vi "mobility_subvi.vi"(0 "Path":path, 9 "NumPts":dbl=5.0, 11 "Row Start":dbl=20.0) -> (1 "Dielectric (d)":dbl, 2 "Capacitance (C)":dbl, 3 "Index":dbl, 4 "XY Graph":cluster{dbl[], dbl[]}[](graph), 6 "Length":dbl, 8 "Vt":dbl, 10 "Width":dbl, 12 "Table Control":string[][](table), 13 "Table Control 2":string[][](table), 14 "Recorded":cluster{"Vt":dbl, "STS":dbl, "On/Off":dbl}, 15 "Mobility":dbl)   [LabVIEW 2011]
uses:
  <vilib>/Utility/file.llb/Read From Spreadsheet File (string).vi
  <vilib>/Analysis/NI_AALPro.lvlib
panel:
  out "Numeric":dbl
  out "String":string
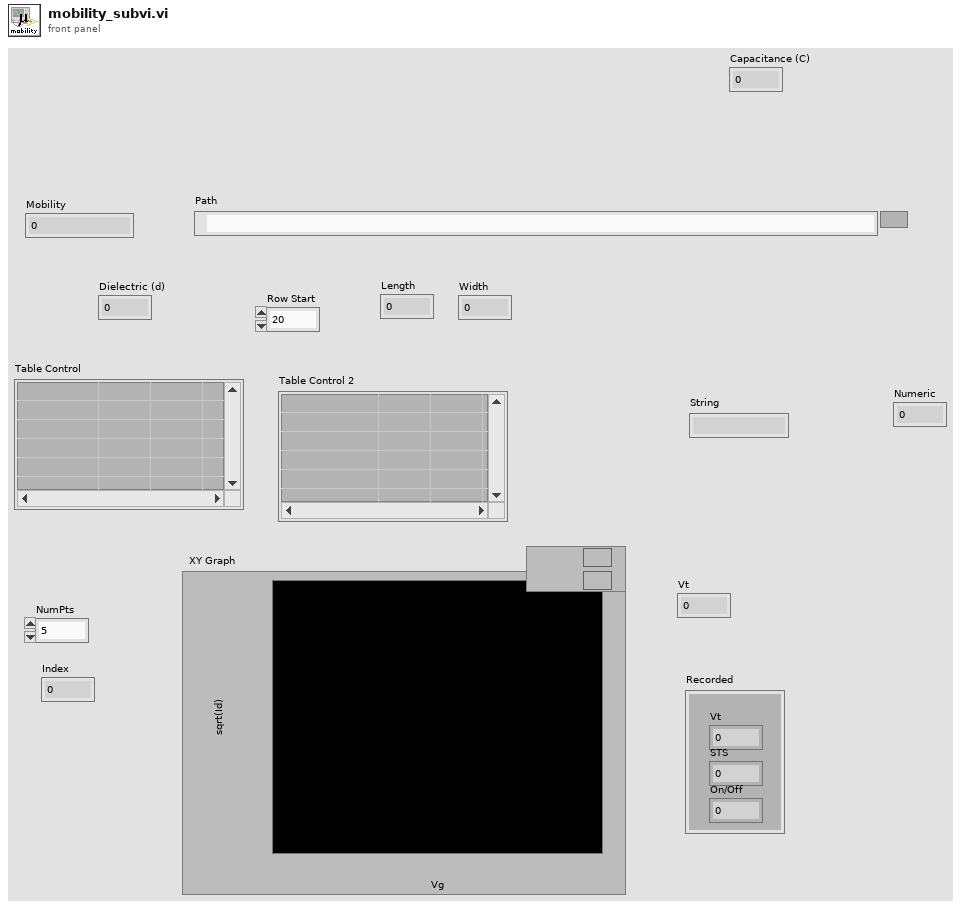
[diagram p1: front panel]
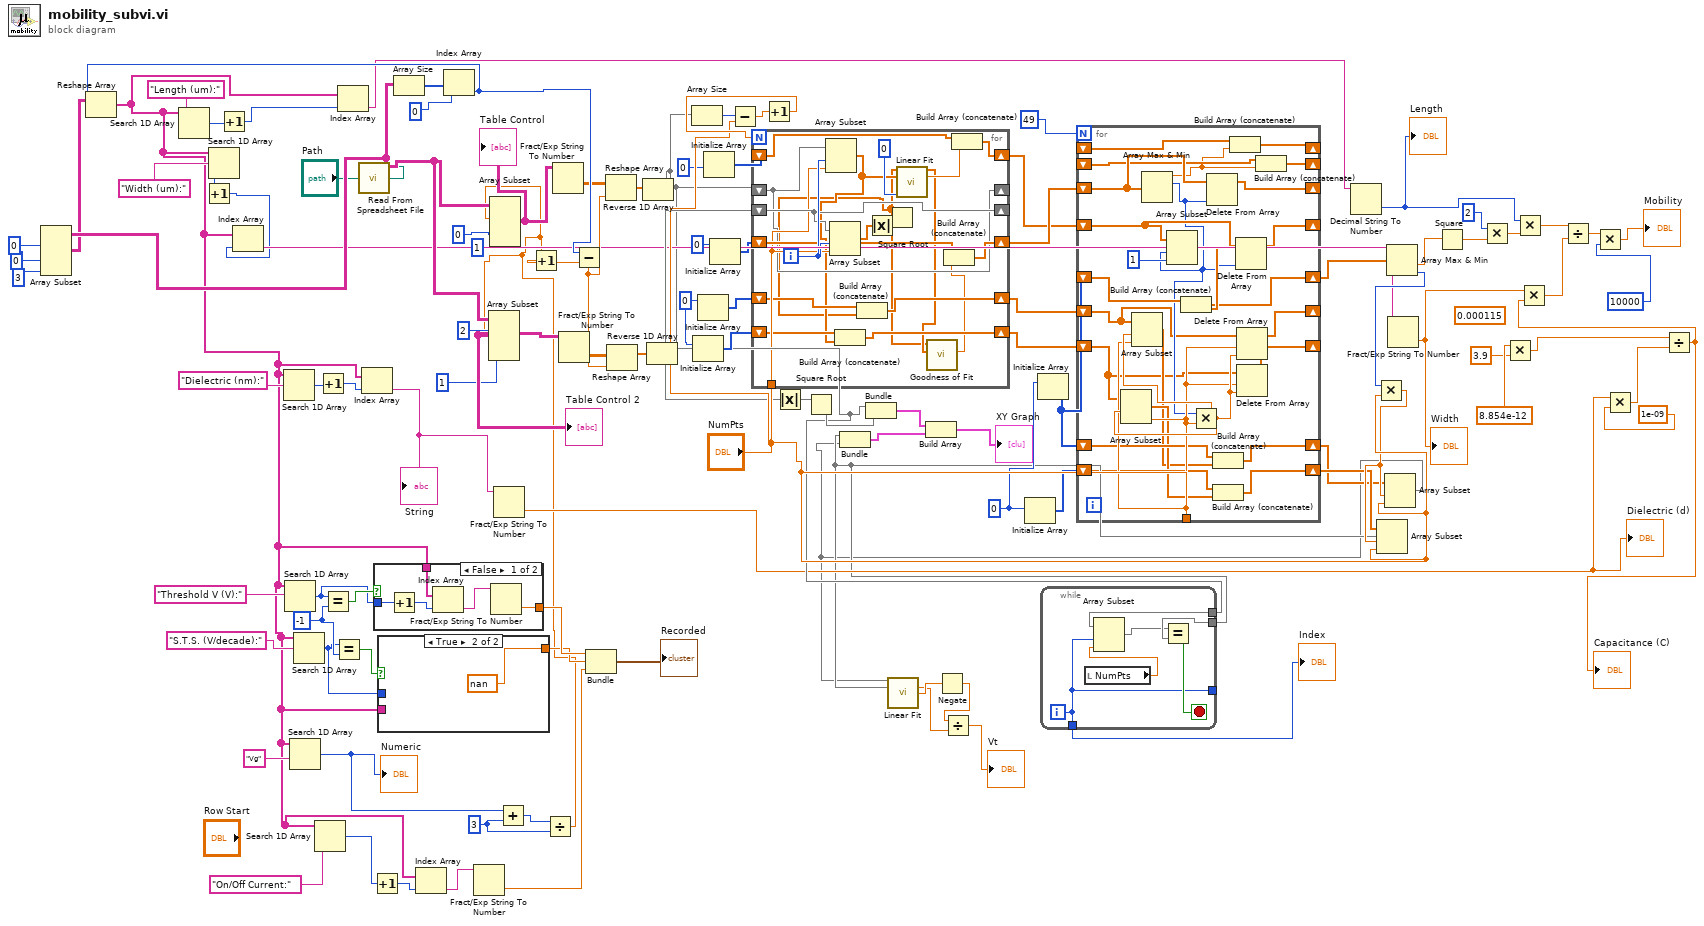
[diagram p0: block diagram]
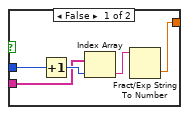
[diagram p2: hidden frame]
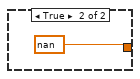
[diagram p3: hidden frame]
diagram:
  w9 = 3
  w20 = -1
  w97 = 0
  w88 = 0
  (unwired) 0.000115
  n1 = call-poly <vilib>:"Read From Spreadsheet File.vi"("file path (dialog if empty)"="Path") -> ("all rows"=w76:string[][])  [unwired: 6 in, 4 out]
  n2 = Array Subset(array=w76, index (row)=0, index (col)=0, length (col)=3) -> (w72:string[][])  [unwired: 1 in]
  n3 = Array Size(array=w76) -> (size(s)=w78:i32[])
  n4 = Index Array(array=w78, index=0) -> (element=w105:i32)
  n5 = Reshape Array(w72, w105) -> (w3:string[])
  n6 = Search 1D Array(1D array=w3, element="Length (um):") -> (index of element=w62:i32)  [unwired: 1 in]
  n7 = Search 1D Array(1D array=w3, element="Width (um):") -> (index of element=w63:i32)  [unwired: 1 in]
  n8 = Increment(x=w63) -> (x+1=w69:i32)
  n9 = Increment(x=w62) -> (x+1=w66:i32)
  n10 = Index Array(array=w3, index=w69) -> (element=w70:string)
  n11 = Search 1D Array(1D array=w3, element="Dielectric (nm):") -> (index of element=w32:i32)  [unwired: 1 in]
  n12 = Search 1D Array(1D array=w3, element="Threshold V (V):") -> (index of element=w17:i32)  [unwired: 1 in]
  n13 = Search 1D Array(1D array=w3, element="Vg") -> (index of element=w11:i32)  [unwired: 1 in]
  "Numeric" <- w11
  n14 = Search 1D Array(1D array=w3, element="S.T.S. (V/decade):") -> (index of element=w16:i32)  [unwired: 1 in]
  n15 = Search 1D Array(1D array=w3, element="On/Off Current:") -> (index of element=w4:i32)  [unwired: 1 in]
  n16 = Increment(x=w32) -> (x+1=w31:i32)
  n17 = Equal?(x=w17, y=w20) -> (x = y?=w19:bool)
  n18 = Equal?(x=w16, y=w20) -> (x = y?=w18:bool)
  n19 = Index Array(array=w3, index=w66) -> (element=w67:string)
  n20 = Index Array(array=w3, index=w31) -> (element=w30:string)
  "String" <- w30
  n21 = Increment(x=w4) -> (x+1=w5:i32)
  n22 = case shown="False" w19 {
    tunnel: w17 -> [w114 _]
    tunnel: w3 -> [w113 _]
    tunnel: [w111 nan] -> w15
    frame False {
      n23 = Increment(x=w114) -> (x+1=w115:i32)
      n24 = Index Array(array=w113, index=w115) -> (element=w112:string)
      n25 = Fract/Exp String To Number(string=w112) -> (number=w111:dbl)  [unwired: 3 in, 1 out]
    }
    frame True {
    }
  }
  n26 = case shown="True" w18 {
    tunnel: w16 -> [w120 _]
    tunnel: w3 -> [w119 _]
    tunnel: [w117 nan] -> w14
    frame False {
      n27 = Increment(x=w120) -> (x+1=w121:i32)
      n28 = Index Array(array=w119, index=w121) -> (element=w118:string)
      n29 = Fract/Exp String To Number(string=w118) -> (number=w117:dbl)  [unwired: 3 in, 1 out]
    }
    frame True {
    }
  }
  n30 = Index Array(array=w3, index=w5) -> (element=w6:string)
  n31 = Fract/Exp String To Number(string=w6) -> (number=w2:dbl)  [unwired: 3 in, 1 out]
  n32 = Fract/Exp String To Number(string=w30) -> (number=w29:dbl)  [unwired: 3 in, 1 out]
  "Dielectric (d)" <- w29
  n33 = Add(x=w11, y=w9) -> (x+y=w10:i32)
  n34 = Divide(x=w10, y=w9) -> (x/y=w8:dbl)
  n35 = Array Subset(array=w76, index (row)=w8, index (col)=2, length (col)=1) -> (w55:string[][])  [unwired: 1 in]
  "Table Control 2" <- w55
  n36 = Array Subset(array=w76, index (row)=w8, index (col)=0, length (col)=1) -> (w54:string[][])  [unwired: 1 in]
  "Table Control" <- w54
  n37 = Increment(x=w8) -> (x+1=w106:dbl)
  n38 = Fract/Exp String To Number(string=w54) -> (number=w56:dbl[][])  [unwired: 3 in, 1 out]
  n39 = Fract/Exp String To Number(string=w55) -> (number=w57:dbl[][])  [unwired: 3 in, 1 out]
  n40 = Subtract(x=w105, y=w106) -> (x-y=w107:dbl)
  n41 = Bundle(w15, w14, w2) -> (→"Recorded":cluster{dbl, dbl, dbl})  [unwired: 1 in]
  n42 = Reshape Array(w56, w107) -> (w93:dbl[])
  n43 = Reshape Array(w57, w107) -> (w94:dbl[])
  n44 = Reverse 1D Array(array=w93) -> (reversed array=w35:dbl[])
  n45 = Reverse 1D Array(array=w94) -> (reversed array=w95:dbl[])
  n46 = Array Size(array=w35) -> (size(s)=w48:i32)
  n47 = Initialize Array(w88) -> (w90:i32[])  [unwired: 1 in]
  n48 = Initialize Array(w88) -> (w89:i32[])  [unwired: 1 in]
  n49 = Initialize Array(0) -> (w49:i32[])  [unwired: 1 in]
  n50 = Initialize Array(0) -> (w50:i32[])  [unwired: 1 in]
  n51 = Subtract(x=w48, y="NumPts") -> (x-y=w109:dbl)
  n52 = Increment(x=w109) -> (x+1=w110:dbl)
  n53 = for {
    N: w110 -> [_]
    shift-right: [w127] -> _
    shift-left: w35 -> [w127]
    shift-right: [w136] -> _
    shift-left: w95 -> [w136]
    shift-right: [w140] -> w59
    shift-left: w49 -> [w139]
    shift-right: [w138] -> w79
    shift-left: w50 -> [w137]
    tunnel: "NumPts" -> [w132]
    shift-right: [w130] -> w91
    shift-left: w89 -> [w131]
    shift-right: [w128] -> w92
    shift-left: w90 -> [w129]
    i -> [w142]
    n54 = Array Subset(array=w127, index=w142, length=w132) -> (w126:dbl[])
    n55 = Array Subset(array=w136, index=w142, length=w132) -> (w135:dbl[])
    n56 = Build Array (concatenate)(w129, w126) -> (w128:dbl[])
    n57 = Absolute Value(x=w135) -> (abs(x)=w134:dbl[])
    n58 = Square Root(x=w134) -> (sqrt(x)=w123:dbl[])
    n59 = Build Array (concatenate)(w131, w123) -> (w130:dbl[])
    n60 = call <vilib>:"Linear Fit.vi"("Y"=w123, "X"=w126, "method"=0) -> ("Best Linear Fit"=w125:dbl[], "slope"=w141:dbl)  [unwired: 8 in, 3 out]
    n61 = call <vilib>:"Goodness of Fit.vi"("Best Fit"=w125, "Y"=w123) -> ("R-square"=w124:dbl)  [unwired: 6 in, 3 out]
    n62 = Build Array (concatenate)(w137, w124) -> (w138:dbl[])
    n63 = Build Array (concatenate)(w139, w141) -> (w140:dbl[])
  }
  n64 = Absolute Value(x=w95) -> (abs(x)=w87:dbl[])
  n65 = Square Root(x=w87) -> (sqrt(x)=w104:dbl[])
  n66 = Bundle(w35, w104) -> (w86:cluster{dbl[], dbl[]})  [unwired: 1 in]
  n67 = Initialize Array(w97) -> (w96:i32[])  [unwired: 1 in]
  n68 = Initialize Array(w97) -> (w101:i32[])  [unwired: 1 in]
  n69 = for {
    N: 49 -> [_]
    shift-right: [w167] -> _
    shift-left: w79 -> [w168]
    shift-right: [w147] -> _
    shift-left: w59 -> [w148]
    shift-right: [w164] -> w64
    shift-left: w101 -> [w163]
    shift-right: [w162] -> _
    shift-left: _ -> [w161]
    shift-right: [w160] -> _
    shift-left: _ -> [w159]
    shift-right: [w158] -> _
    shift-left: w91 -> [w144]
    shift-right: [w156] -> _
    shift-left: w92 -> [w143]
    tunnel: "NumPts" -> [w155]
    shift-right: [w154] -> w98
    shift-left: w101 -> [w153]
    shift-right: [w152] -> w99
    shift-left: w96 -> [w151]
    n70 = Array Max & Min(array=w168) -> (max value=w146:dbl, max index (indices)=w145:i32)  [unwired: 2 out]
    n71 = Array Subset(array=w148, index=w145, length=1) -> (w165:dbl[])
    n72 = Build Array (concatenate)(w163, w165) -> (w164:dbl[])
    n73 = Multiply(x=w145, y=w155) -> (x*y=w157:dbl)
    n74 = Array Subset(array=w143, index=w157, length=w155) -> (w150:dbl[])
    n75 = Array Subset(array=w144, index=w157, length=w155) -> (w149:dbl[])
    n76 = Delete From Array(array=w168, index=w145) -> (array with subset deleted=w167:dbl[])  [unwired: 1 in, 1 out]
    n77 = Build Array (concatenate)(w153, w149) -> (w154:dbl[])
    n78 = Build Array (concatenate)(w151, w150) -> (w152:dbl[])
    n79 = Build Array (concatenate)(w161, w146) -> (w162:dbl[])
    n80 = Delete From Array(array=w148, index=w145) -> (array with subset deleted=w147:dbl[])  [unwired: 1 in, 1 out]
    n81 = Delete From Array(array=w144, length=w155, index=w157) -> (array with subset deleted=w158:dbl[])  [unwired: 1 out]
    n82 = Delete From Array(array=w143, length=w155, index=w157) -> (array with subset deleted=w156:dbl[])  [unwired: 1 out]
    n83 = Build Array (concatenate)(w159, w146) -> (w160:dbl[])
  }
  n84 = Decimal String To Number(string=w67) -> (number=w68:i32)  [unwired: 2 in, 1 out]
  "Length" <- w68
  n85 = Array Max & Min(array=w64) -> (min value=w53:dbl, min index (indices)=w100:i32)  [unwired: 2 out]
  n86 = Multiply(x=w100, y="NumPts") -> (x*y=w102:dbl)
  n87 = Array Subset(array=w99, index=w102, length="NumPts") -> (w28:dbl[])
  n88 = while {
    tunnel: [w169] -> _
    tunnel: w35 -> [w173]
    tunnel: w28 -> [w172]
    tunnel: [w169] -> w34
    i -> [w169]
    stop <- w174 stop-if-true
    n89 = local read "NumPts"() -> (w170:dbl)
    n90 = Array Subset(array=w173, index=w169, length=w170) -> (w171:dbl[])
    n91 = Equal?(x=w171, y=w172) -> (x = y?=w174:bool)
  }
  "Index" <- w34
  n92 = Array Subset(array=w98, index=w102, length="NumPts") -> (w27:dbl[])
  n93 = Bundle(w28, w27) -> (w103:cluster{dbl[], dbl[]})  [unwired: 1 in]
  n94 = call <vilib>:"Linear Fit.vi"("Y"=w27, "X"=w28) -> ("slope"=w24:dbl, "intercept"=w26:dbl)  [unwired: 9 in, 3 out]
  n95 = Build Array(w86, w103) -> (→"XY Graph":cluster{dbl[], dbl[]}[])
  n96 = Negate(x=w26) -> (-x=w25:dbl)
  n97 = Divide(x=w25, y=w24) -> (x/y=→"Vt":dbl)
  n98 = Fract/Exp String To Number(string=w70) -> (number=w71:dbl)  [unwired: 3 in, 1 out]
  "Width" <- w71
  n99 = Square(x=w53) -> (x^2=w47:dbl)
  n100 = Multiply(x=2, y=w47) -> (x*y=w46:dbl)
  n101 = Multiply(x=8.854e-12, y=3.9) -> (x*y=w84:dbl)
  n102 = Multiply(x=w68, y=w46) -> (x*y=w45:dbl)
  n103 = Multiply(x=w29, y=1e-09) -> (x*y=w83:dbl)
  n104 = Divide(x=w84, y=w83) -> (x/y=w1:dbl)
  "Capacitance (C)" <- w1
  n105 = Multiply(x=w71, y=w1) -> (x*y=w44:dbl)
  n106 = Divide(x=w45, y=w44) -> (x/y=w42:dbl)
  n107 = Multiply(x=w42, y=10000) -> (x*y=→"Mobility":dbl)
